vi "Vorticity.vi"(4 "vort max":dbl(slide)=2929.2929292929293 scale=0.0..5000.0, 6 "vort min val":dbl, 7 "step vort":i32, 8 "Values":T1, 9 "Mean/Median":u16(ring) items=["Median", "Mean"], 10 "AVG #":i32=3 min=1, 11 "Vector out":csg[][](array[numeric])) -> (0 "markervlas":cluster{"vort max":dbl, u32}[](array[cluster]), 1 "vorticity rad/s":dbl[][](graph), 2 "KE":dbl[][](array[numeric]), 5 "EL mW/m":dbl[][](graph))   [LabVIEW 2022 SP3]
uses:
  VPIParams.ctl
panel:
  in  "x":sgl=1.0
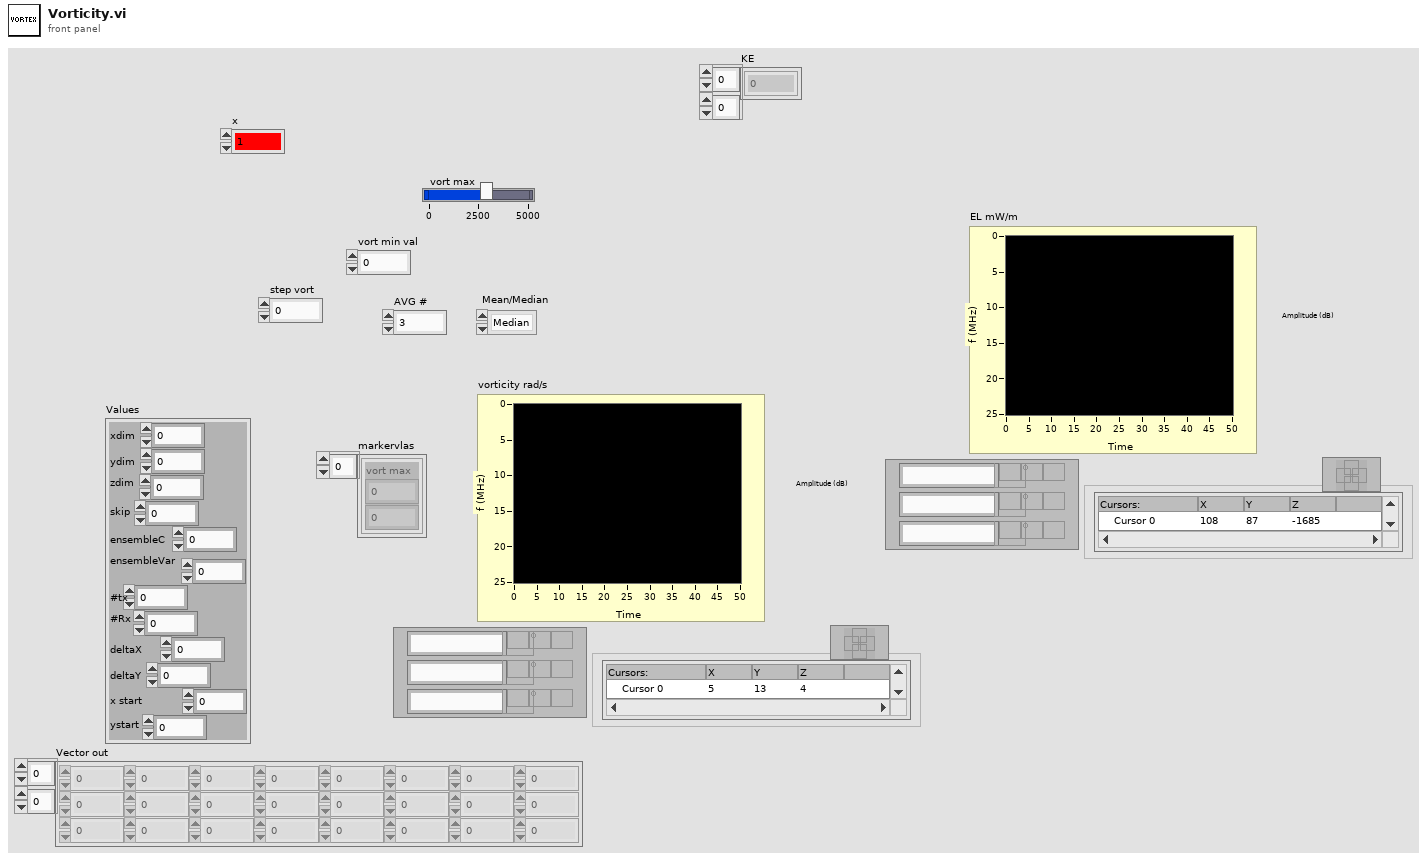
[diagram p1: front panel]
types:
  T1 = typedef "VPIParams.ctl" = cluster{"xdim":dbl, "ydim":dbl, "zdim":dbl, "skip":dbl, "ensembleC":dbl, "ensembleVar\n":dbl, "#tx":dbl, "#Rx":dbl, "deltaX":dbl, "deltaY":dbl, "x start":dbl, "ystart":dbl}
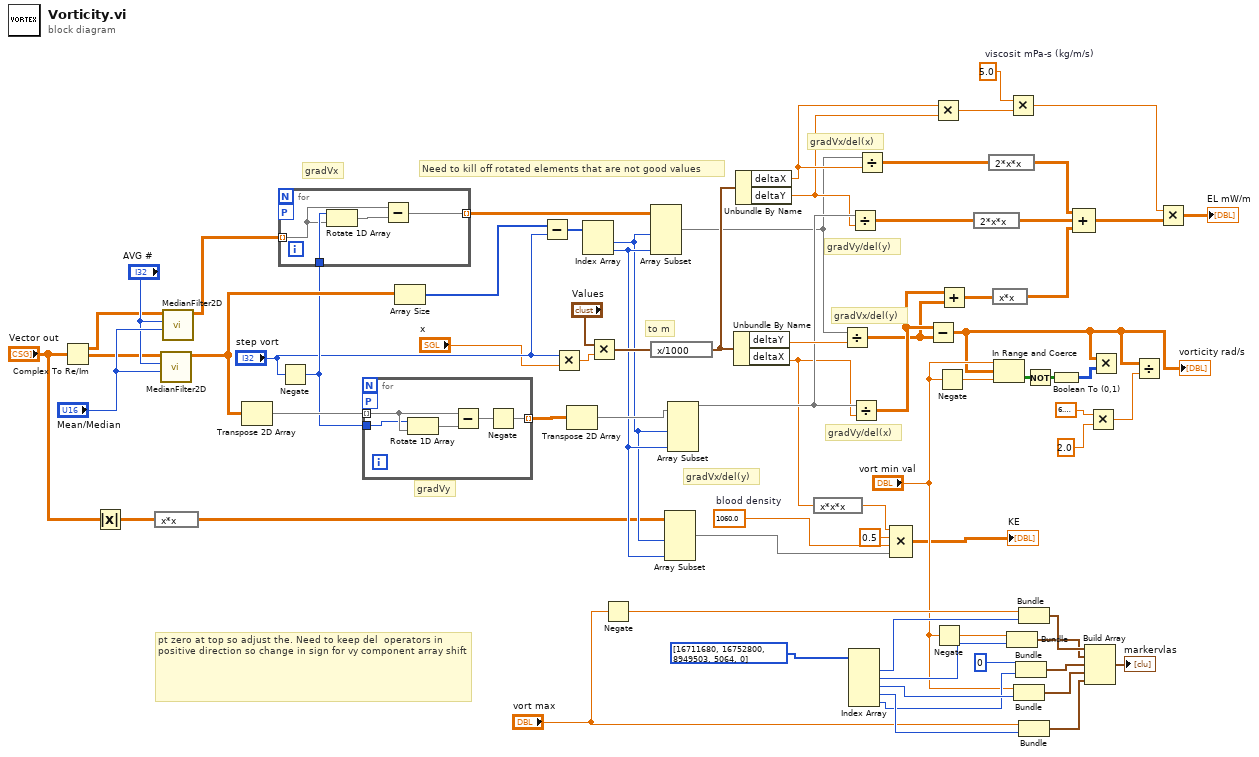
[diagram p0: block diagram]
diagram:
  w6 = 1060.0  # blood density
  w17 = 5.0  # viscosit mPa-s (kg/m/s)
  # "gradVx"
  # "gradVy"
  # "gradVx/del(x)"
  # "gradVy/del(y)"
  # "gradVx/del(y)"
  # "Need to kill off rotated elements that are not good values"
  # "gradVx/del(y)"
  # "gradVy/del(x)"
  # "pt zero at top so adjust the. Need to keep del  operators in positive direction so change in sign for vy component array shift"
  # "to m"
  n1 = Complex To Re/Im(x + iy="Vector out") -> (x=w38:sgl[][], y=w48:sgl[][])
  n2 = Absolute Value(x="Vector out") -> (abs(x)=w14:sgl[][])
  n3 = expression code="x*x"(w14) -> (w11:sgl[][])
  n4 = call "MedianFilter2D.vi"("Operation"="Mean/Median", "Pts to use"="AVG #", "Raw In"=w48) -> ("output array"=w44:sgl[][])  [unwired: 8 in]
  n5 = call "MedianFilter2D.vi"("Operation"="Mean/Median", "Pts to use"="AVG #", "Raw In"=w38) -> ("output array"=w45:sgl[][])  [unwired: 8 in]
  n6 = Transpose 2D Array(2D array=w44) -> (transposed array=w73:sgl[][])
  n7 = Negate(x="step vort") -> (-x=w39:i32)
  n8 = for {
    tunnel: w45 -> [w75] mode=indexing
    tunnel: [w74] -> w43 mode=indexing
    tunnel: w39 -> [w76]
    workers-P: _ -> [_]
    n9 = Rotate 1D Array(1:w75, 2:w76) -> (0:w77:sgl[])
    n10 = Subtract(x=w75, y=w77) -> (x-y=w74:sgl[])
  }
  n11 = for {
    tunnel: w73 -> [w81] mode=indexing
    tunnel: [w78] -> w46 mode=indexing
    tunnel: w39 -> [w80]
    workers-P: _ -> [_]
    n12 = Rotate 1D Array(1:w81, 2:w80) -> (0:w82:sgl[])
    n13 = Subtract(x=w81, y=w82) -> (x-y=w79:sgl[])
    n14 = Negate(x=w79) -> (-x=w78:sgl[])
  }
  n15 = Array Size(array=w44) -> (size(s)=w41:i32[])
  n16 = Subtract(x=w41, y="step vort") -> (x-y=w40:i32[])
  n17 = Multiply(x="step vort", y="x") -> (x*y=w36:sgl)
  n18 = Transpose 2D Array(2D array=w46) -> (transposed array=w42:sgl[][])
  n19 = Index Array(array=w40) -> (element #1=w12:i32, element #2=w13:i32)  [unwired: 2 in]
  n20 = Multiply(x="Values", y=w36) -> (x*y=w32:T1)
  n21 = Negate(x="vort max") -> (-x=w61:dbl)
  n22 = Array Subset(array=w43, length (row)=w12, length (col)=w13) -> (w16:sgl[][])  [unwired: 2 in]
  n23 = expression code="x/1000"(w32) -> (w30:T1)
  n24 = Array Subset(array=w11, length (row)=w12, length (col)=w13) -> (w7:sgl[][])  [unwired: 2 in]
  n25 = Array Subset(array=w42, length (row)=w12, length (col)=w13) -> (w29:sgl[][])  [unwired: 2 in]
  n26 = Unbundle By Name(w30) -> ("deltaY"=w31:dbl, "deltaX"=w10:dbl)
  n27 = Unbundle By Name(w30) -> ("deltaX"=w23:dbl, "deltaY"=w22:dbl)
  n28 = expression code="x*x*x"(w10) -> (w9:dbl)
  n29 = Divide(x=w16, y=w31) -> (x/y=w33:dbl[][])
  n30 = Index Array(array=u32[] [16711680, 16752800, 8949503, 5064, 0]) -> (element #1=w67:u32, element #2=w66:u32, element #3=w65:u32, element #4=w64:u32, element #5=w58:u32)  [unwired: 5 in]
  n31 = Divide(x=w29, y=w22) -> (x/y=w27:dbl[][])
  n32 = Divide(x=w29, y=w10) -> (x/y=w34:dbl[][])
  n33 = Divide(x=w16, y=w23) -> (x/y=w28:dbl[][])
  n34 = Compound Arithmetic op=MULTIPLY(w9, 0.5 ("value"), w6, w7) -> (→"KE":dbl[][])
  n35 = Subtract(x=w34, y=w33) -> (x-y=w1:dbl[][])
  "vorticity rad/s" <- w1
  n36 = Multiply(x=w23, y=w22) -> (x*y=w19:dbl)
  n37 = Negate(x="vort min val") -> (-x=w57:dbl)
  n38 = Negate(x="vort min val") -> (-x=w72:dbl)
  n39 = Add(x=w34, y=w33) -> (x+y=w51:dbl[][])
  n40 = expression code="2*x*x"(w27) -> (w25:dbl[][])
  n41 = expression code="2*x*x"(w28) -> (w24:dbl[][])
  n42 = expression code="x*x"(w51) -> (w26:dbl[][])
  n43 = In Range and Coerce(upper limit="vort min val", x=w1, lower limit=w72) -> (In Range?=w71:bool[][])  [unwired: 1 out]
  n44 = Bundle(w57, w66) -> (w62:cluster{dbl, u32})  [unwired: 1 in]
  n45 = Multiply(x=w17, y=w19) -> (x*y=w18:dbl)
  n46 = Bundle("vort min val"="vort min val", w65) -> (w54:cluster{"vort min val":dbl, u32})  [unwired: 1 in]
  n47 = Bundle(0, w58) -> (w56:cluster{i32, u32})  [unwired: 1 in]
  n48 = Bundle(w61, w67) -> (w63:cluster{dbl, u32})  [unwired: 1 in]
  n49 = Bundle("vort max"="vort max", w64) -> (w55:cluster{"vort max":dbl, u32})  [unwired: 1 in]
  n50 = Not(x=w71) -> (.not. x?=w69:bool[][])
  n51 = Boolean To (0,1)(Boolean=w69) -> (0, 1=w70:i16[][])
  n52 = Compound Arithmetic op=ADD(w24, w25, w26) -> (w21:dbl[][])
  n53 = Build Array(w63, w62, w56, w54, w55) -> (→"markervlas":cluster{"vort max":dbl, u32}[])
  n54 = Multiply(x=6.283185307179586, y=2.0) -> (x*y=w2:dbl)
  n55 = Multiply(x=w1, y=w70) -> ()  [unwired: 1 out]
  n56 = Divide(x=w1, y=w2) -> ()  [unwired: 1 out]
  n57 = Multiply(x=w18, y=w21) -> (x*y=→"EL mW/m":dbl[][])
